vi "Test Ignore Test Case With No Child Items.vi"(8 "error in (no error)":errorcluster, 11 "Result Model Tests in":refnum<class "Result Model Test Enumeration.lvclass">) -> (0 "error out":errorcluster, 3 "Result Model Tests out":refnum<class "Result Model Test Enumeration.lvclass">)   [LabVIEW 2020, in "Result Model Test Enumeration.lvclass"]
uses:
  Result Model Test Enumeration.lvclass
  C:/Program Files (x86)/National Instruments/LabVIEW 2020/vi.lib/Astemes/LUnit/Core/LUnit Test Case/Test Case.lvclass
  <vilib>/Astemes/LUnit/Core/LUnit Test Case/Test Case.lvclass/Test Case.ctl
  206db1ee-aa99-40b9-8881-171f2a77c34b.vi
  <vilib>/Astemes/LUnit/Core/LUnit Test Case/Private/Append Pass Result.vi
  <vilib>/Astemes/LUnit/Core/LUnit Test Case/Private/Append Fail Result.vi
  206db1ee-aa99-40b9-8881-171f2a77c34b.vi/9c5d11cd-9439-4240-a1ee-d9baace9c924.vi
  <vilib>/Astemes/LUnit/Core/LUnit Test Case/Private/Run In UI.vi
  <vilib>/Utility/error.llb/Clear Errors.vi
  source/User Interface/Result Model by Reference/Result Model by Reference.lvclass
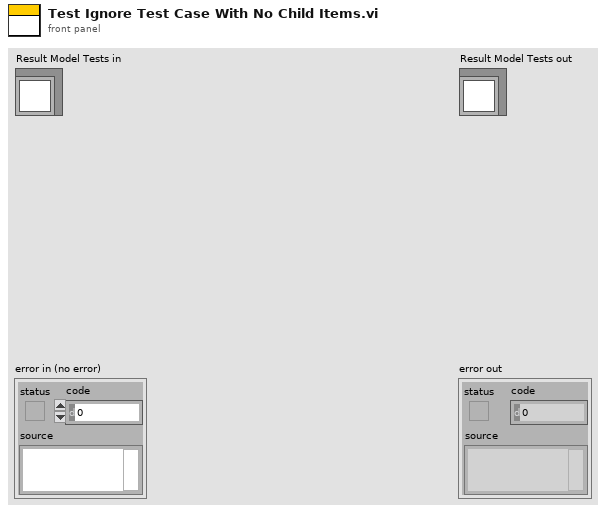
[diagram p1: front panel]
types:
  T1 = cluster{"Left Cell String":string, "Child Text":string[], "Child Tag":string, "Item Indent":i32, "Child Only?":bool, "Glyph Index":i32}[]
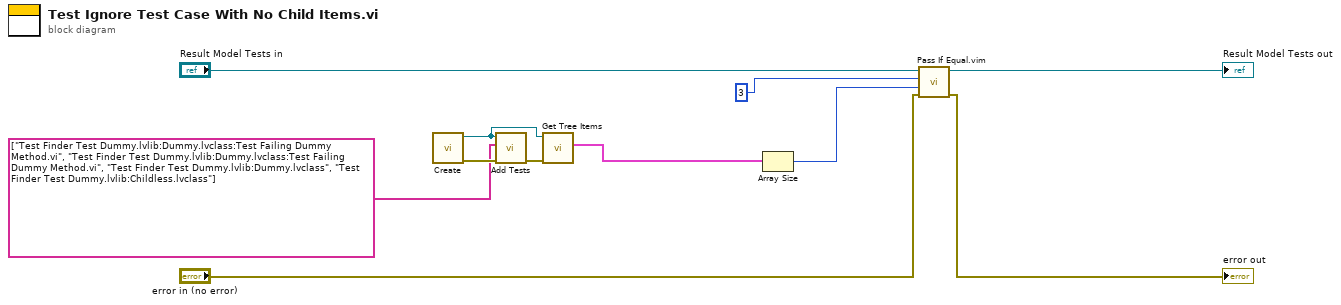
[diagram p0: block diagram]
diagram:
  n1 = call "Create.vi"() -> ("error out"=w6:errorcluster, "Result Model out"=w4:refnum<class "Result Model by Reference.lvclass">)  [unwired: 10 in]
  n2 = call "Add Tests.vi"("error in (no error)"=w6, "Tests"=string[] ["Test Finder Test Dummy.lvlib:Dummy.lvclass:Test Failing Dummy Method.vi", "Test Finder Test Dummy.lvlib:Dummy.lvclass:Test Failing Dummy Method.vi", "Test Finder Test Dummy.lvlib:Dummy.lvclass", "Test Finder Test Dummy.lvlib:Childless.lvclass"] ("Array"), "Result Model by Reference In"=w4) -> ("error out"=w5:errorcluster)  [unwired: 8 in]
  n3 = call "Get Tree Items.vi"("error in (no error)"=w5, "Result Model by Reference In"=w4) -> ("Tree Items"=w3:T1)  [unwired: 8 in, 1 out]
  n4 = Array Size(array=w3) -> (size(s)=w2:i32)
  n5 = call "Pass If Equal.vim"("error in (no error)"="error in (no error)", "Actual"=w2, "Expected"=3 ("Item Indent"), "LUnit Test Case In"="Result Model Tests in") -> ("error out"=→"error out":errorcluster, "LUnit Test Case Out"=→"Result Model Tests out":refnum<class "Result Model Test Enumeration.lvclass">)  [unwired: 6 in]
